vi "OpenSpace.vi"() -> ()   [LabVIEW 2016]
panel:
  in  "WindowsMediaPlayer":refnum<k7>(container)
  in  "Previous Button":bool
  # "Open Space"
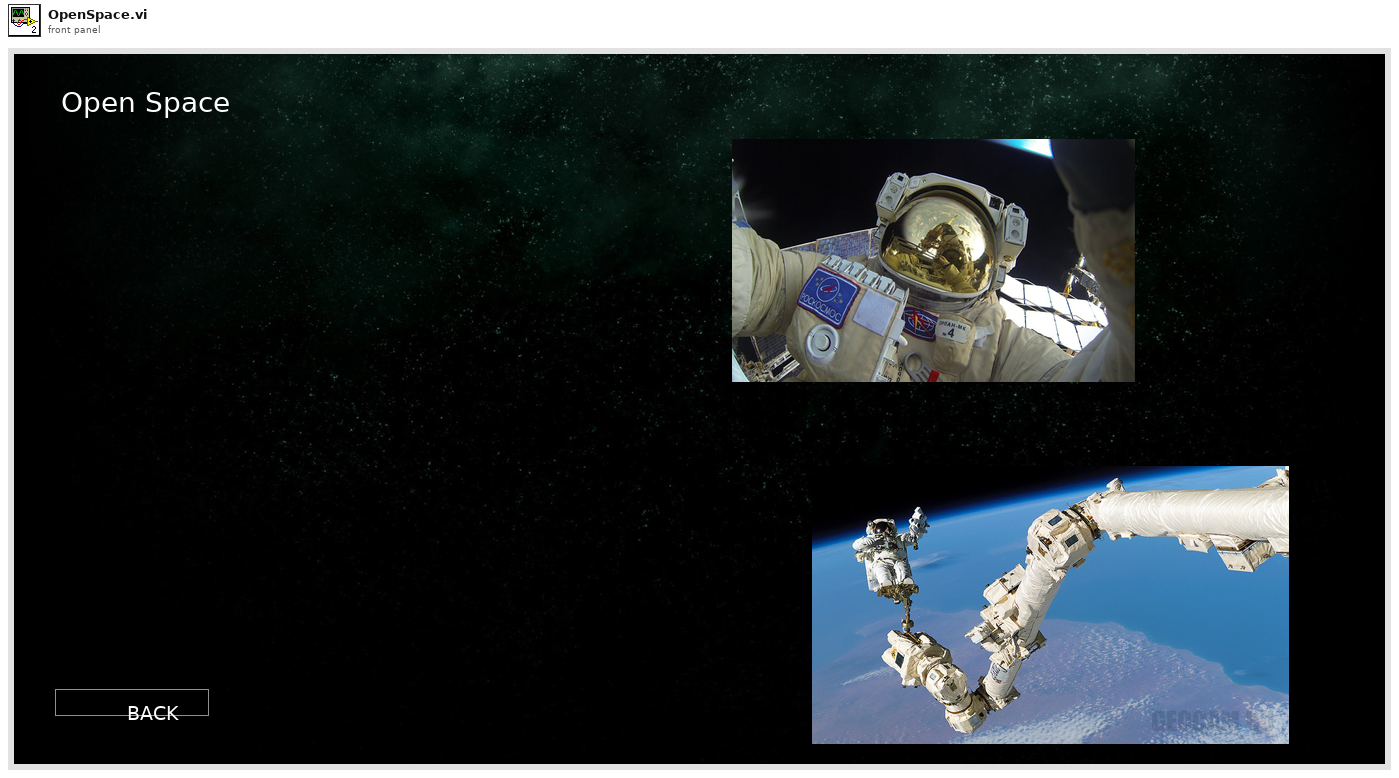
[diagram p1: front panel]
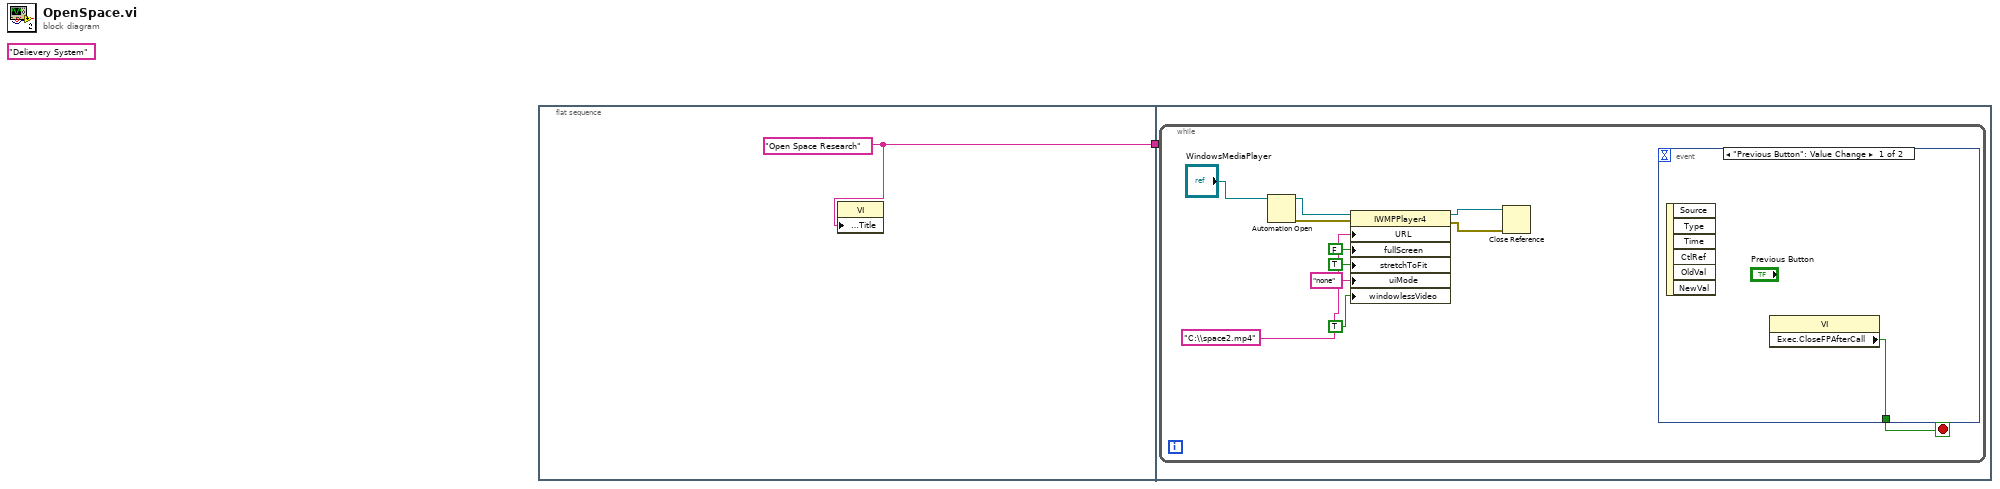
[diagram p0: block diagram]
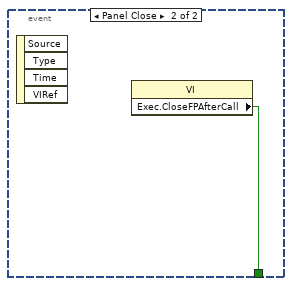
[diagram p2: hidden frame]
diagram:
  (unwired) "Delievery System" ("Front Panel Window:Title")
  n1 = flat-sequence {
    tunnel: [w2] -> w1
    tunnel: w1 -> [_]
    frame #0 {
      w2 = "Open Space Research" ("Front Panel Window:Title")
      n2 = property class="VI"("Front Panel.Title"=w2) -> ()  [unwired: 2 in, 2 out]
    }
    frame #1 {
      n3 = while {
        stop <- w13 stop-if-true
        n4 = Automation Open(Automation Refnum="WindowsMediaPlayer") -> (Automation Refnum=w12:refnum<k7>, error out=w11:errorcluster)  [unwired: 3 in]
        n5 = property class="IWMPPlayer4"(reference=w12, error in=w11, "URL"="C:\\space2.mp4", "fullScreen"=FALSE, "stretchToFit"=TRUE, "uiMode"="none", "windowlessVideo"=TRUE) -> (reference out=w10:refnum<k7>, error out=w9:errorcluster)
        n6 = Close Reference(reference=w10, error in (no error)=w9) -> ()  [unwired: 1 out]
        n7 = event shown="[0] \"Previous Button\": Value Change" {
          selector: _ -> [_ _]
          dyn-events: _ -> [_ _]
          timeout: _ -> [_ _]
          tunnel: [w14 w15] -> w13
          event "Previous Button": Value Change {
            n8 = event-data() -> ()  [unwired: 1 in, 6 out]
            n9 = property class="VI"() -> ("Exec.CloseFPAfterCall"=w14:bool)  [unwired: 2 in, 2 out]
          }
          event Panel Close {
            n10 = event-data() -> ()  [unwired: 1 in, 4 out]
            n11 = property class="VI"() -> ("Exec.CloseFPAfterCall"=w15:bool)  [unwired: 2 in, 2 out]
          }
        }
      }
    }
  }
